vi "Configure Decimator 1.vi"(5 "lock-in.decimator1 0":enum16{"None", "FIR", "SOS"}(ring), 8 "error in (no error)":errorcluster, 9 "lock-in.decimation1 0":i32, 11 "LIA Host Interface in":refnum<class "LIA Host Interface.lvclass">) -> (0 "error out":errorcluster, 3 "LIA Host Interface out":refnum<class "LIA Host Interface.lvclass">)   [LabVIEW 2018, in "LIA Debugging.lvclass"]
uses:
  LIA Debugging.lvclass
  Shared/lib/interface/Interface/LIA Host Interface.lvclass
  Shared/lib/interface/Interface FPGA/LIA Host Interface FPGA.lvclass
  Shared/lib/interface/Interface FPGA/Properties/FpgaSession_GET.vi
  <vilib>/Utility/error.llb/Error Cluster From Error Code.vi
  <vilib>/rvi/errors/niLvFpgaAdjustHostInterfaceError.vi
  <vilib>/rvi/interface/nirviReadWriteControl/nirviReadWriteControl.xnode
  NiFpgaLv.dll
  <vilib>/rvi/interface/Simulation/niFpgaSimulationCallBeginRW.vi
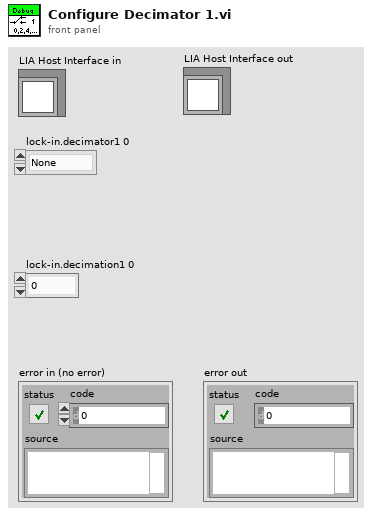
[diagram p1: front panel]
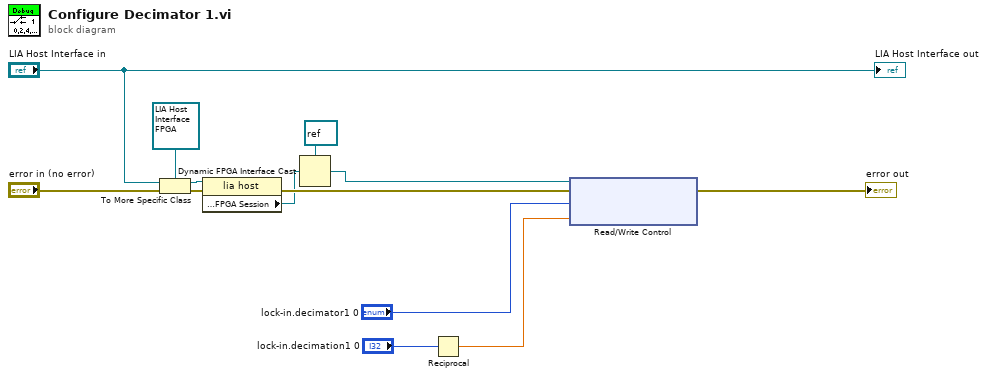
[diagram p0: block diagram]
diagram:
  n1 = To More Specific Class(target class=refnum<class "LIA Host Interface FPGA.lvclass"> refnum ("lia host"), reference="LIA Host Interface in", error in="error in (no error)") -> (specific class reference=w9:refnum<class "LIA Host Interface FPGA.lvclass">, error out=w8:errorcluster)
  n2 = property class="lia host"(reference=w9, error in=w8) -> (error out=w13:errorcluster, "Properties:FPGA Session"=w10:refnum<k20>)  [unwired: 1 out]
  n3 = Dynamic FPGA Interface Cast(Session In=refnum<k20> refnum ("fpga type"), Type=w10) -> (Session Out=w4:refnum<k20>)
  n4 = Reciprocal(x="lock-in.decimation1 0") -> (1/x=w3:dbl)
  n5 = xnode "Read/Write Control"("FPGA VI Reference In"=w4, "error in"=w13, "lock-in.decimator1 0"="lock-in.decimator1 0", "lock-in.fir1 fs 0"=w3) -> ("error out"=→"error out":errorcluster)  [unwired: 1 out]
  "LIA Host Interface out" <- "LIA Host Interface in"
